vi "Test_LogIfError_WarningFlagged_WarningLogged.vi"(8 "error in (no error)":errorcluster, 11 "TestCase in":refnum<class "TestLocalLogInstance.lvclass">) -> (0 "error out":errorcluster, 3 "TestCase out":refnum<class "TestLocalLogInstance.lvclass">)   [LabVIEW 2017, in "TestLocalLogInstance.lvclass"]
uses:
  TestLocalLogInstance.lvclass
  Source/Composed Log/Types/Log Level.ctl
  Source/Composed Log/LoggerReference/LoggerReference.lvclass/LoggerReference.ctl
  Source/LVQueue Sink/LVQueue Sink.lvclass/LVQueue Sink.ctl
  d39b0a5b-172c-4f26-bba3-73eadbc629b5.vi
  Source/Composed Log/LoggerReference/Return Aggregate Queues.vi
  Source/Composed Log/LoggerReference/Add Aggregate Log.vi
  d39b0a5b-172c-4f26-bba3-73eadbc629b5.vi/720e5afd-0a00-437c-9ba6-379bbfc37dba.vi
  Source/Composed Log/LoggerReference/Send Add Sink.vi
  Source/LVQueue Sink/LVQueue Sink.lvclass
  C:/CS/Internal/LabVIEW/Logger/Source/Composed Log/Log Sink/Log Sink.lvclass
  Source/Composed Log/Application Logger/Launch Worker Loop.vi
  Source/Composed Log/LoggerReference/Initialize Logger Instance.vi
  Source/Composed Log/LoggerReference/LoggerReference.lvclass
  Source/Composed Log/IErrorFormat/IErrorFormat.lvclass
  Source/Composed Log/Log Sink/Log Sink.lvclass
  <vilib>/addons/_JKI Toolkits/VI Tester/TestCase.llb/TestCase.lvclass
  Source/Composed Log/Composed Log.lvlib
  C:/Program Files (x86)/National Instruments/LabVIEW 2017/vi.lib/addons/_JKI Toolkits/VI Tester/TestCase.llb/TestCase.lvclass
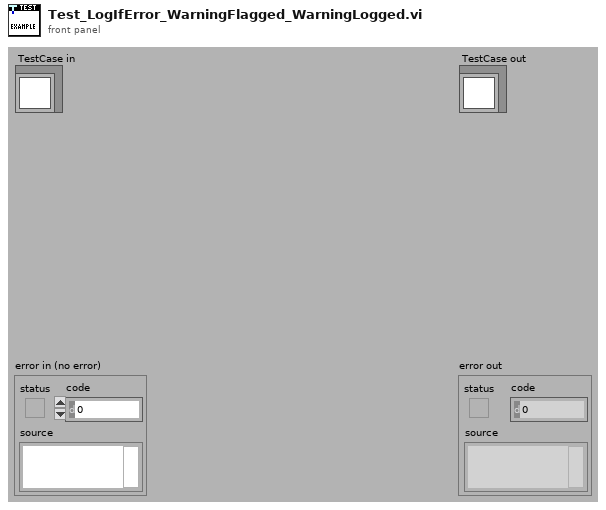
[diagram p1: front panel]
types:
  T1 = typedef "Composed Log.lvlib/Log Level.ctl" = enum16{"Debug", "Info", "Warning", "Error", "Critical"}
  T2 = typedef "Composed Log.lvlib/Log Packet.ctl" = cluster{"Data To Log":string, "Source":string, "Event Level":T1, "Event Time":timestamp}
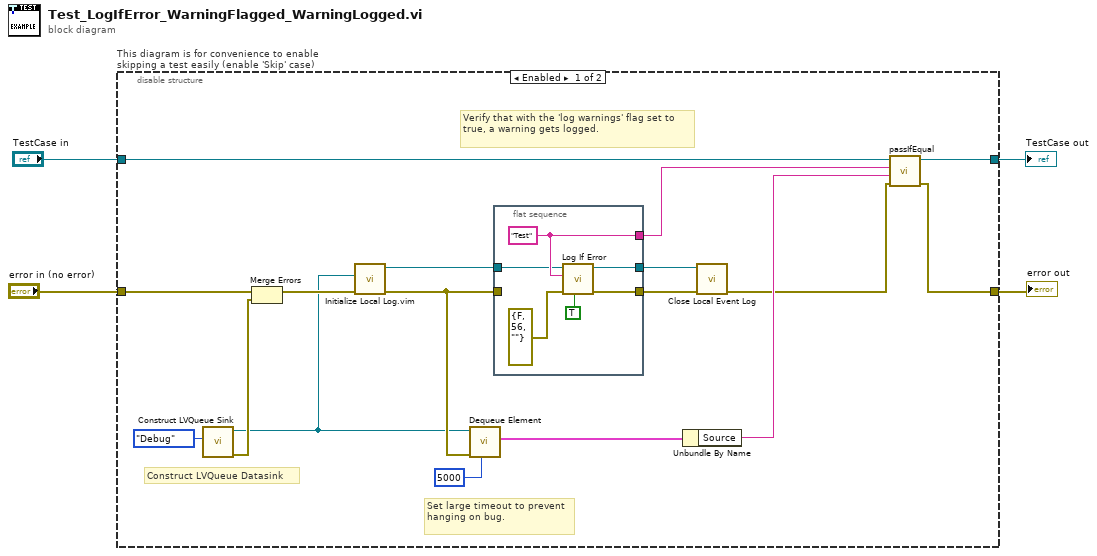
[diagram p0: block diagram]
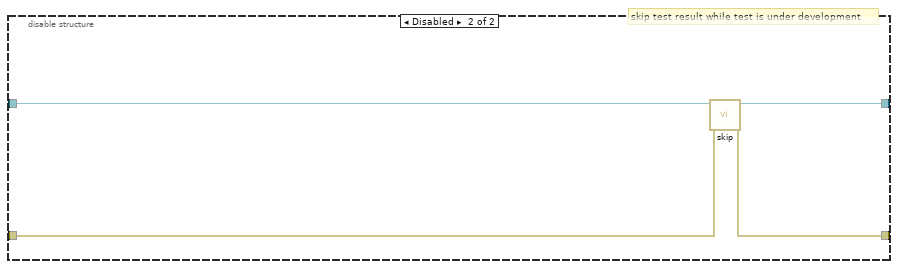
[diagram p2: hidden frame]
diagram:
  n1 = disable-structure "This diagram is for convenience to enable skipping a test easily (enable 'Skip' case)" shown="Enabled" {
    disable-tunnel: "TestCase in" -> [w15 w31]
    disable-tunnel: [w14 w29] -> w1
    disable-tunnel: [w16 w30] -> w3
    disable-tunnel: "error in (no error)" -> [w21 w28]
    frame Enabled {
      # "Construct LVQueue Datasink"
      # "Set large timeout to prevent hanging on bug."
      # "Verify that with the 'log warnings' flag set to true, a warning gets logged."
      n2 = call "Construct LVQueue Sink.vi"("LogLevel"=Log_Level."Debug") -> ("error out"=w17:errorcluster, "LVQueue Sink out"=w7:refnum<class "LVQueue Sink.lvclass">)  [unwired: 9 in]
      n3 = Merge Errors(w21, w17) -> (w9:errorcluster)
      n4 = call "Initialize Local Log.vim"("error in (no error)"=w9, "Startup Sink(s)"=w7) -> ("error out"=w8:errorcluster, "Log Instance Reference"=w6:refnum<class "LoggerReference.lvclass">)  [unwired: 7 in, 1 out]
      n5 = call "Dequeue Element.vi"("timeout in ms (-1)"=5000, "error in (no error)"=w8, "LVQueue Sink in"=w7) -> ("Log Packet"=w18:T2)  [unwired: 5 in, 3 out]
      n6 = flat-sequence {
        tunnel: w8 -> [_]
        tunnel: [w27] -> w11
        tunnel: [w24] -> w12
        tunnel: w6 -> [w23]
        tunnel: [w22] -> w5
        frame #0 {
          w24 = "Test" ("SourceID")
          n7 = call "Log If Error.vi"("Include Warnings(F)"=TRUE, "Error In"=errorcluster {"status"=FALSE, "code"=56, "source"=""}, "SourceID"=w24, "Log Instance"=w23) -> ("error out"=w27:errorcluster, "Log Instance Out"=w22:refnum<class "LoggerReference.lvclass">)  [unwired: 6 in]
        }
      }
      n8 = Unbundle By Name(w18) -> ("Source"=w13:string)
      n9 = call "Close Local Event Log.vi"("error in (no error)"=w11, "Log Instance"=w5) -> ("error out"=w10:errorcluster)  [unwired: 9 in]
      n10 = call-dynamic "passIfEqual.vi"("error in (no error)"=w10, "y"=w13, "x"=w12, "TestCase in"=w15) -> ("error out"=w16:errorcluster, "TestCase out"=w14:refnum<class "TestLocalLogInstance.lvclass">)  [unwired: 6 in]
    }
    frame Disabled {
      # "skip test result while test is under development"
      n11 = call <vilib>:"skip.vi"("error in (no error)"=w28, "TestCase in"=w31) -> ("error out"=w30:errorcluster, "TestCase out"=w29:refnum<class "TestLocalLogInstance.lvclass">)  [unwired: 8 in]
    }
  }
  "error out" <- w3
  "TestCase out" <- w1
